vi "Simple Spectrum Analyzer (sim).vi"() -> ()   [LabVIEW 2023]
doc: "Constructs a simple Spectrum Analyzer example using the Waveform Measurement VIs. This example simulates a waveform, and computes the averaged, windowed power spectrum. The VI graphs the power spectrum in the desired units."
uses:
  <vilib>/measure/maspectr.llb/FFT Power Spectrum and PSD for 1 Chan.vi
  <vilib>/measure/NI_MAPro.lvlib
panel:
  in  "window":i32(ring) items=["Rectangle", "Hanning", "Hamming", "Blackman-Harris", "Exact Blackman", "Blackman", "Flat Top", "4 Term B-Harris ", "7 Term B-Harris", "Low Sidelobe", "Blackman Nuttall", "Triangle", "Bartlett-Hanning", "Bohman", "Parzen", "Welch", "Kaiser", "Dolph-Chebyshev", "Gaussian"]
  in  "resolution (# of lines)":u32=800
  out "sampling info":cluster{"Fs":dbl, "#s":dbl} {"#s" format="%#.6g"; "Fs" format="%#.6g"}
  out "FFT info":T1 {"FFT resolution (Hz)" format="%#.6g"; "Record Length" format="%#.6g"}
  in  "y scale":enum16{"Linear", "dB"}(ring)=enum."dB"
  in  "Restart averaging":bool
  in  "baseband span":dbl=10000.0 format="%#.6g"
  in  "Stop":bool
  out "Spectrum":cluster{"f0":dbl, "df":dbl, "Y":dbl[]}(graph)
  in  "averaging parameters":T2={"averaging mode"=enum."RMS averaging", "weighting mode"=enum."Exponential", "number of averages"=10} {"number of averages" min=1}
  out "averages completed":dbl
  out "Linear averaging done":bool
  # "Overview: Demonstrates use of the FFT Power Spectrum and PSD VI to window a signal and display the averaged power spectrum.\nRequirements: LabVIEW Full Development System\nInstructions: \n1. Run the VI.\n2. Change the baseband span, resolution, and y scale, and note the resulting Spectrum graph and FFT info values.\n3. Change the averaging parameters to explore various FFT averaging and weighting modes.\n4. Click Stop to stop the VI."
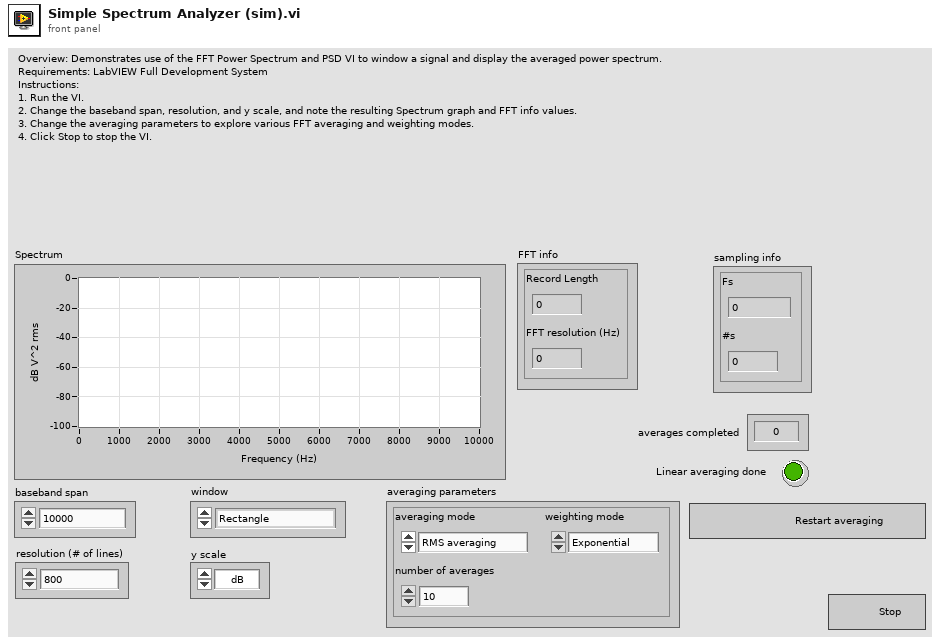
[diagram p1: front panel]
types:
  T1 = cluster{"Record Length":dbl, "FFT resolution (Hz)":dbl}
  T2 = cluster{"averaging mode":enum16{"No averaging", "Vector averaging", "RMS averaging", "Peak hold"}, "weighting mode":enum16{"Linear", "Exponential"}, "number of averages":u32}
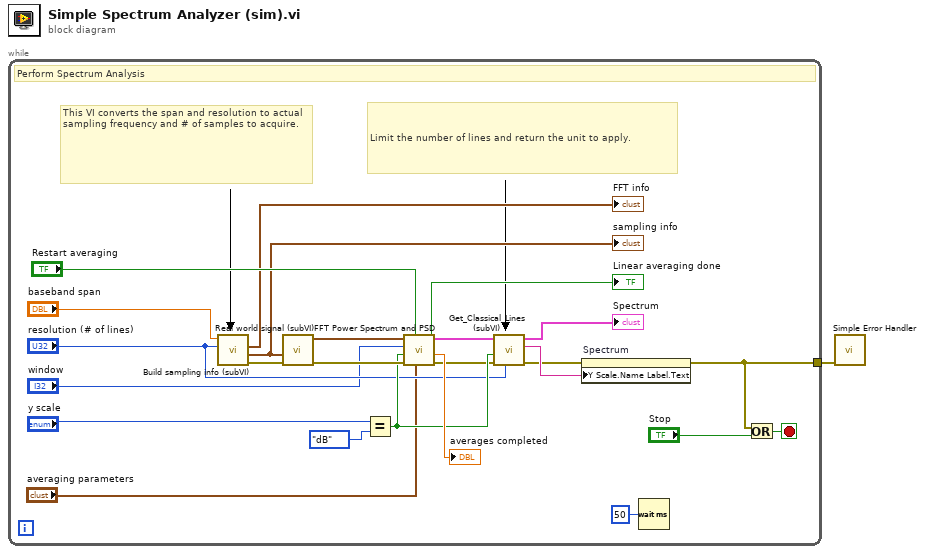
[diagram p0: block diagram]
diagram:
  n1 = while {
    tunnel: [w4] -> w1
    stop <- w18 stop-if-true
    # "Limit the number of lines and return the unit to apply."
    # "This VI converts the span and resolution to actual sampling frequency and # of samples to acquire."
    # "Perform Spectrum Analysis"
    n2 = call "Build sampling info (subVI).vi"("resolution (# of lines)"="resolution (# of lines)", "baseband span"="baseband span") -> ("error out"=w21:errorcluster, "sampling info"=w6:cluster{"Fs":dbl, "#s":dbl}, "FFT info"=→"FFT info":T1)  [unwired: 7 in]
    "sampling info" <- w6
    n3 = call "Real world signal (subVI).vi"("error in (no error)"=w21, "sampling info"=w6) -> ("error out"=w14:errorcluster, "time signal"=w15:waveform(dbl))  [unwired: 8 in]
    n4 = Equal?(x="y scale", y=enum16{"Linear", "dB"}."dB" ("Display")) -> (x = y?=w13:bool)
    n5 = call-poly <vilib>:"FFT Power Spectrum and PSD.vi"("averaging parameters"="averaging parameters", "restart averaging (F)"="Restart averaging", "error in (no error)"=w14, "dB On (F)"=w13, "window"="window", "time signal"=w15) -> ("error out"=w12:errorcluster, "averages completed"=→"averages completed":dbl, "averaging done"=→"Linear averaging done":bool, "Power Spectrum / PSD"=w11:cluster{"f0":dbl, "df":dbl, "magnitude":dbl[]})  [unwired: 2 in]
    n6 = call "Get_Classical_Lines (subVI).vi"("resolution (# of lines)"="resolution (# of lines)", "error in (no error)"=w12, "dB On (F)"=w13, "power spectrum"=w11) -> ("error out"=w5:errorcluster, "Unit"=w10:string, "spectral lines"=→"Spectrum":cluster{"f0":dbl, "df":dbl, "Y":dbl[]})  [unwired: 5 in]
    n7 = property on="Spectrum" class="WFGraph (strict)"(error in=w5, "Y Scale.Name Label.Text"=w10) -> (error out=w4:errorcluster)  [unwired: 1 in, 1 out]
    n8 = Wait (ms)(milliseconds to wait=u32 50 ("millisecond multiple")) -> ()  [unwired: 1 out]
    n9 = Or(x=w4, y="Stop") -> (x .or. y?=w18:bool)
  }
  n10 = call <vilib>:"Simple Error Handler.vi"("error in (no error)"=w1) -> ()  [unwired: 4 in, 5 out]
